vi "Configure Multi Eval Meas Limit Emission Mask.vi"(0 "VISA resource name":refnum<visa-resource-name>, 1 "Enable (On)":bool=TRUE, 2 "Frequency End (0Hz)":dbl format="%#.9p", 3 "RBW (1 MHz)":i32(ring) items=["1 MHz"], 5 "Instance (1)":T3=1, 7 "Area (1)":T2=1, 9 "Bandwidth (50 MHz)":T1 items=["50 MHz", "100 MHz", "200 MHz", "400 MHz"], 11 "error in (no error)":errorcluster, 12 "Frequency Start (0Hz)":dbl format="%#.9p", 13 "Level (0.0)":dbl format="%^.3e") -> (4 "VISA resource name out":refnum<visa-resource-name>, 15 "error out":errorcluster)   [LabVIEW 2015, in "Rohde&Schwarz CMXP NR FR2 Measurement.lvlib"]
doc: "Defines general requirements for the emission mask area number <area>. The activation state, the area borders, an upper limit and the resolution bandwidth must be specified.\nThe emission mask applies to the channel bandwidth <bw>.\n\nAttribute:\nRSCMXPNRFR2M_ATTR_MULTI_EVAL_MEASUREMENT_LIMIT_EMISSION_MASK\n\nRemote-control command:\nCONFigure:NRMMw:MEAS<i>:MEValuation:LIMit:SEMask:AREA<area>:CBANdwidth<bw>"
uses:
  <instrlib>/Rohde&Schwarz CMXP NR FR2 Measurement/Rohde&Schwarz CMXP NR FR2 Measurement.lvlib
  <instrlib>/Rohde&Schwarz CMXP NR FR2 Measurement/Private/_Instance.ctl
  <instrlib>/Rohde&Schwarz CMXP NR FR2 Measurement/Private/_Area.ctl
  <instrlib>/Rohde&Schwarz CMXP NR FR2 Measurement/Private/_Bandwidth.ctl
  <instrlib>/Rohde&Schwarz CMXP NR FR2 Measurement/Private/rsidr_core.llb/rsidr_core.lvlib
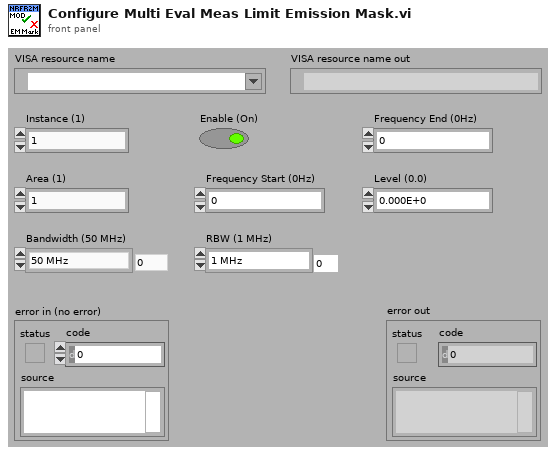
[diagram p1: front panel]
types:
  T1 = typedef "Rohde&Schwarz CMXP NR FR2 Measurement.lvlib/_Bandwidth.ctl" = i32
  T2 = typedef "Rohde&Schwarz CMXP NR FR2 Measurement.lvlib/_Area.ctl" = i32
  T3 = typedef "Rohde&Schwarz CMXP NR FR2 Measurement.lvlib/_Instance.ctl" = i32
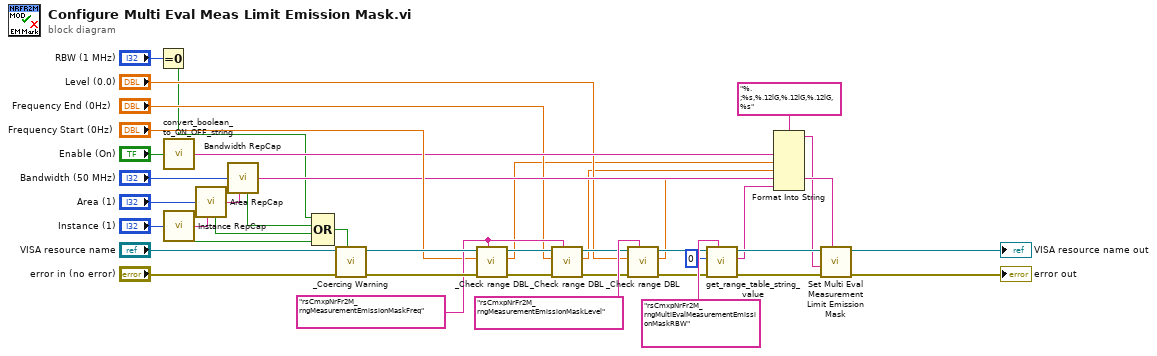
[diagram p0: block diagram]
diagram:
  w29 = "rsCmxpNrFr2M_rngMeasurementEmissionMaskFreq"
  n1 = Equal To 0?(x="RBW (1 MHz)") -> (x = 0?=w4:bool)
  n2 = call <instrlib>:"convert_boolean_to_ON_OFF_string.vi"("boolean value in"="Enable (On)") -> ("string value out"=w16:string)  [unwired: 4 in]
  n3 = call <instrlib>:"Instance RepCap.vi"("Instance In"="Instance (1)") -> ("In Range?"=w36:bool, "RepCap Identifier Out"=w2:string)  [unwired: 1 in]
  n4 = call <instrlib>:"Area RepCap.vi"("SEM Area In"="Area (1)", "RepCap String In (\"\")"=w2) -> ("In Range?"=w35:bool, "RepCap Identifier Out"=w34:string)
  n5 = call <instrlib>:"Bandwidth RepCap.vi"("Bandwidth In"="Bandwidth (50 MHz)", "RepCap String In (\"\")"=w34) -> ("In Range?"=w33:bool, "RepCap Identifier Out"=w15:string)
  n6 = Compound Arithmetic op=OR(w4, w33, w35, w36) -> (w38:bool)
  n7 = call <instrlib>:"_Coercing Warning.vi"("In Range?"=w38, "error in (no error)"="error in (no error)", "VISA resource name"="VISA resource name") -> ("error out"=w31:errorcluster, "VISA resource name out"=w30:refnum<visa-resource-name>)  [unwired: 7 in]
  n8 = call <instrlib>:"_Check range DBL.vi"("Range Table Identifier"=w29, "error in (no error)"=w31, "DBL Value In"="Frequency Start (0Hz)", "VISA resource name"=w30) -> ("error out"=w27:errorcluster, "DBL Value Out"=w8:dbl, "VISA resource name out"=w28:refnum<visa-resource-name>)  [unwired: 5 in]
  n9 = call <instrlib>:"_Check range DBL.vi"("Range Table Identifier"=w29, "error in (no error)"=w27, "DBL Value In"="Frequency End (0Hz)", "VISA resource name"=w28) -> ("error out"=w21:errorcluster, "DBL Value Out"=w7:dbl, "VISA resource name out"=w22:refnum<visa-resource-name>)  [unwired: 5 in]
  n10 = call <instrlib>:"_Check range DBL.vi"("Range Table Identifier"="rsCmxpNrFr2M_rngMeasurementEmissionMaskLevel", "error in (no error)"=w21, "DBL Value In"="Level (0.0)", "VISA resource name"=w22) -> ("error out"=w20:errorcluster, "DBL Value Out"=w6:dbl, "VISA resource name out"=w19:refnum<visa-resource-name>)  [unwired: 5 in]
  n11 = call <instrlib>:"get_range_table_string_value.vi"("Range Table ID in"="rsCmxpNrFr2M_rngMultiEvalMeasurementEmissionMaskRBW", "error in"=w20, "I32 input"=0, "VISA resource name"=w19) -> ("error out"=w13:errorcluster, "String Value out"=w5:string, "VISA resource name out"=w14:refnum<visa-resource-name>)  [unwired: 5 in]
  n12 = Format Into String(format string="%.;%s,%.12lG,%.12lG,%.12lG,%s", w16, w8, w7, w6, w5) -> (resulting string=w1:string)  [unwired: 2 in, 1 out]
  n13 = call "Set Multi Eval Measurement Limit Emission Mask"("Repeated Capabilities"=w15, "error in (no error)"=w13, "Multi Eval Measurement Limit Emission Mask ()"=w1, "instrument handle"=w14) -> ("error out"=→"error out":errorcluster, "instrument handle out"=→"VISA resource name out":refnum<visa-resource-name>)  [unwired: 6 in]
